vi "Teleop - Rev Change Check (SubVI).vi"(10 "controlPanelPosition PID":T1, 11 "Trigger Output":bool) -> (3 "Changed?":bool)   [LabVIEW 2019]
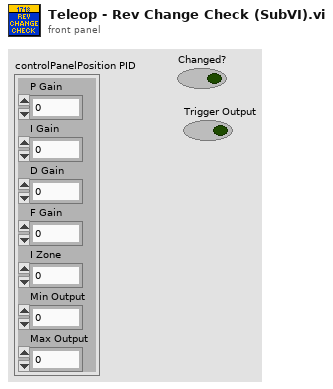
[diagram p1: front panel]
types:
  T1 = cluster{"P Gain":dbl, "I Gain":dbl, "D Gain":dbl, "F Gain":dbl, "I Zone":dbl, "Min Output":dbl, "Max Output":dbl}
  T2 = cluster{"P Gain":bool, "I Gain":bool, "D Gain":bool, "F Gain":bool, "I Zone":bool, "Min Output":bool, "Max Output":bool}
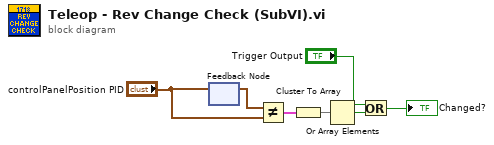
[diagram p0: block diagram]
diagram:
  n1 = feedback #1() -> (w4:T1)  [unwired: 1 in]
  n2 = feedback-in #1("controlPanelPosition PID") -> ()
  n3 = Not Equal?(x=w4, y="controlPanelPosition PID") -> (x != y?=w6:T2)
  n4 = Cluster To Array(cluster=w6) -> (array=w5:bool[])
  n5 = Or Array Elements(Boolean array=w5) -> (logical OR=w1:bool)
  n6 = Or(x="Trigger Output", y=w1) -> (x .or. y?=→"Changed?":bool)
